vi "Save-images.vi"(8 "error in":errorcluster, 10 "Storage element in":T1 {"Temperature characteristics"."Stand. dev. temperature" format="%#.1f"; "Temperature characteristics"."Min. temperature" format="%#.0f"; "Temperature characteristics"."Max. temperature" format="%#.0f"; "Temperature characteristics"."Average temperature" format="%#.0f"}, 11 "Storage params. ref.":refnum<data-value>) -> (0 "error IO":errorcluster, 2 "Storage element":T1 {"Temperature characteristics"."Stand. dev. temperature" format="%#.1f"; "Temperature characteristics"."Min. temperature" format="%#.0f"; "Temperature characteristics"."Max. temperature" format="%#.0f"; "Temperature characteristics"."Average temperature" format="%#.0f"}, 3 "Storage params. ref.":refnum<data-value>)   [LabVIEW 2013, in "CameraVision.lvlib" / "CV-Main.lvclass"]
uses:
  CV-Main.lvclass
  Storage/CV-Storage.lvclass
  Buffers/Storage-buffer.ctl
  <vilib>/vision/Image Controls.llb/IMAQ Image.ctl
  Temperature/Temperature-characteristics.ctl
  Analysis/Characteristics-cluster.ctl
  Storage/CV-Storage.lvclass/CV-Storage.ctl
  Storage/Read Storage directory.vi
  Storage/Read Save what.vi
  Storage/Read Storage labels.vi
  Storage/Read Storage prefix.vi
  Storage/Read Image file type.vi
  Storage/Read Camera suffix.vi
  Storage/Save-image-with-right-filetype.vi
  Temperature/CV-Temperature.lvclass
  Analysis/CV-Analysis.lvclass
  Buffers/CV-Buffers.lvclass
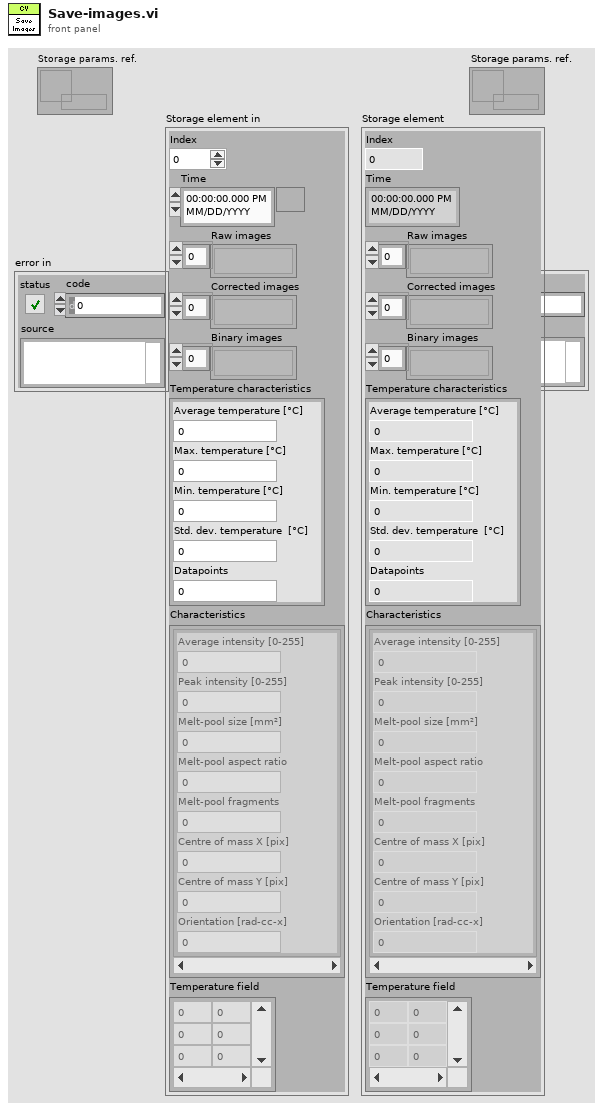
[diagram p1: front panel]
types:
  T1 = typedef "CameraVision.lvlib/CV-Buffers.lvclass/Storage-buffer.ctl" = cluster{"Index":i32, "Time":timestamp, "Raw images":T2[], "Corrected images":T2[], "Binary images":T2[], "Temperature characteristics":T3, "Characteristics":T4[], "Temperature field":dbl[][]}
  T2 = typedef "IMAQ Image.ctl" = refnum<image>
  T3 = typedef "CameraVision.lvlib/CV-Temperature.lvclass/Temperature-characteristics.ctl" = cluster{"Average temperature ":dbl, "Max. temperature":dbl, "Min. temperature":dbl, "Stand. dev. temperature":dbl, "Datapoints":dbl}
  T4 = typedef "CameraVision.lvlib/CV-Analysis.lvclass/Characteristics-cluster.ctl" = cluster{"Average intensity":dbl, "Peak intensity":dbl, "Melt-pool size":dbl, "Melt-pool aspect ratio":dbl, "Melt-pool fragments":dbl, "Centre of mass X":dbl, "Centre of mass Y":dbl, "Orientation":dbl}
  T5 = cluster{"Original":bool, "Corrected":bool, "Binary":bool, "Temperature":bool, "Characteristics":bool, "Mapping":bool, "TemperatureValues":bool}
  T6 = typedef "CameraVision.lvlib/Storage.lvclass/Storage-types-labels.ctl" = cluster{"Original":string, "Corrected":string, "Binary":string, "Temperature":string, "Characteristics":string, "Mapping":string, "TemperatureValues":string}
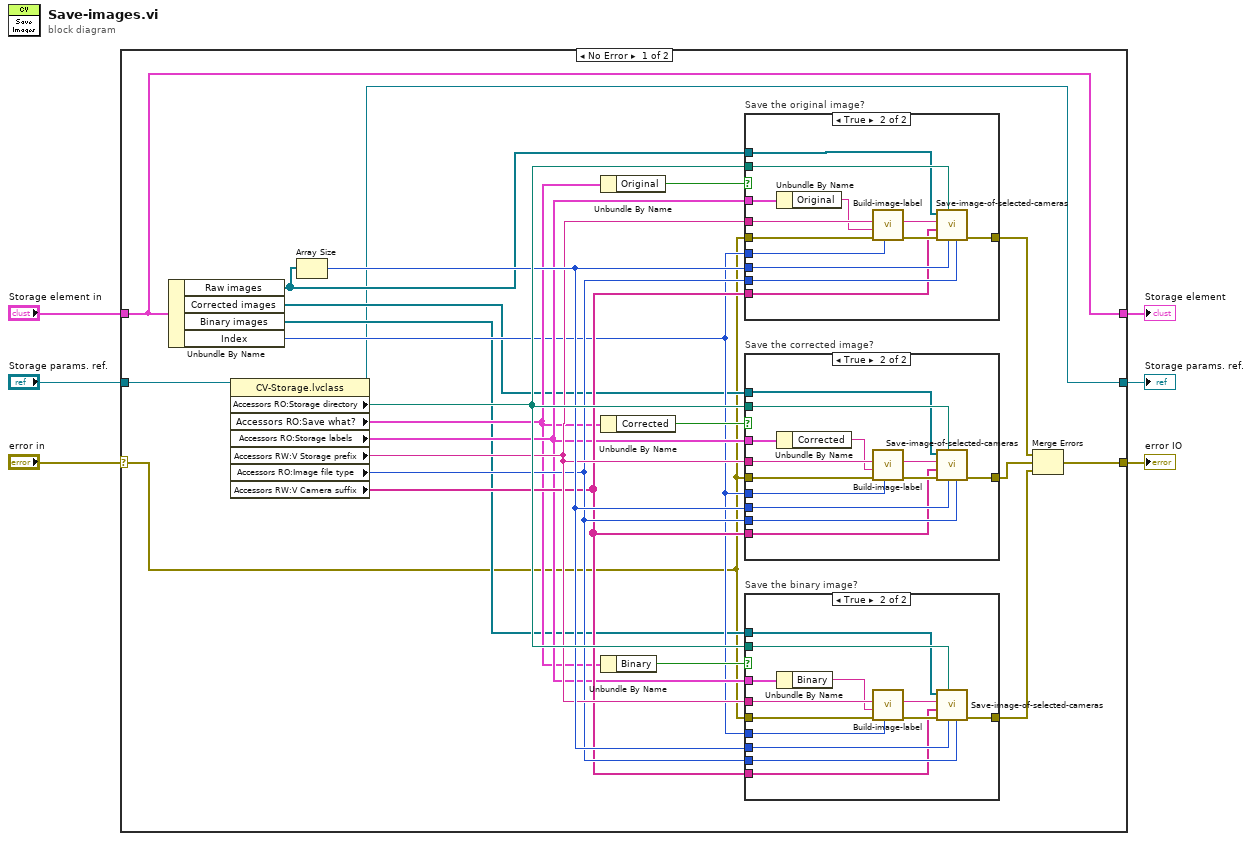
[diagram p0: block diagram]
diagram:
  n1 = case shown="No Error" "error in" {
    selector: "error in" -> [w11 w73]
    tunnel: [w7 w73] -> w6
    tunnel: "Storage params. ref." -> [w25 w72]
    tunnel: "Storage element in" -> [w9 w71]
    tunnel: [w9 w71] -> w2
    tunnel: [w8 w72] -> w1
    frame No Error {
      n2 = Unbundle By Name(w9) -> ("Raw images"=w10:T2[], "Corrected images"=w12:T2[], "Binary images"=w13:T2[], "Index"=w14:i32)
      n3 = property class="CV-Storage.lvclass"(reference=w25) -> (reference out=w8:refnum<data-value>, "Accessors RO:Storage directory"=w28:path, "Accessors RO:Save what?"=w21:T5, "Accessors RO:Storage labels"=w22:T6, "Accessors RW:V Storage prefix"=w26:string, "Accessors RO:Image file type"=w24:enum16{"JPG", "BMP", "PNG"}, "Accessors RW:V Camera suffix"=w23:string[])  [unwired: 1 in, 1 out]
      n4 = Array Size(array=w10) -> (size(s)=w27:i32)
      n5 = Unbundle By Name(w21) -> ("Original"=w20:bool)
      n6 = Unbundle By Name(w21) -> ("Corrected"=w19:bool)
      n7 = Unbundle By Name(w21) -> ("Binary"=w18:bool)
      n8 = case "Save the original image?" shown="True" w20 {
        tunnel: w14 -> [_ w62]
        tunnel: w11 -> [w57 w64]
        tunnel: w10 -> [_ w58]
        tunnel: w28 -> [_ w68]
        tunnel: w27 -> [_ w63]
        tunnel: w26 -> [_ w67]
        tunnel: w22 -> [_ w66]
        tunnel: w24 -> [_ w61]
        tunnel: w23 -> [_ w60]
        tunnel: [w57 w59] -> w17
        frame False {
        }
        frame True {
          n9 = Unbundle By Name(w66) -> ("Original"=w65:string)
          n10 = call "Build-image-label.vi"("Image #"=w62, "error in"=w64, "Image label"=w65, "Base file name"=w67) -> ("error IO"=w69:errorcluster, "Filename"=w70:string)  [unwired: 6 in]
          n11 = call "Save-image-of-selected-cameras.vi"("Image file type"=w61, "Cameras"=w63, "Storage directory"=w68, "error in"=w69, "Camera suffix"=w60, "Filename"=w70, "Image references"=w58) -> ("error IO"=w59:errorcluster)  [unwired: 4 in]
        }
      }
      n12 = case "Save the corrected image?" shown="True" w19 {
        tunnel: w14 -> [_ w48]
        tunnel: w11 -> [w43 w50]
        tunnel: w12 -> [_ w44]
        tunnel: w28 -> [_ w54]
        tunnel: w27 -> [_ w49]
        tunnel: w26 -> [_ w53]
        tunnel: w22 -> [_ w52]
        tunnel: w24 -> [_ w47]
        tunnel: w23 -> [_ w46]
        tunnel: [w43 w45] -> w16
        frame False {
        }
        frame True {
          n13 = Unbundle By Name(w52) -> ("Corrected"=w51:string)
          n14 = call "Build-image-label.vi"("Image #"=w48, "error in"=w50, "Image label"=w51, "Base file name"=w53) -> ("error IO"=w55:errorcluster, "Filename"=w56:string)  [unwired: 6 in]
          n15 = call "Save-image-of-selected-cameras.vi"("Image file type"=w47, "Cameras"=w49, "Storage directory"=w54, "error in"=w55, "Camera suffix"=w46, "Filename"=w56, "Image references"=w44) -> ("error IO"=w45:errorcluster)  [unwired: 4 in]
        }
      }
      n16 = case "Save the binary image?" shown="True" w18 {
        tunnel: w14 -> [_ w34]
        tunnel: w11 -> [w29 w36]
        tunnel: w13 -> [_ w30]
        tunnel: w28 -> [_ w40]
        tunnel: w27 -> [_ w35]
        tunnel: w26 -> [_ w39]
        tunnel: w22 -> [_ w38]
        tunnel: w24 -> [_ w33]
        tunnel: w23 -> [_ w32]
        tunnel: [w29 w31] -> w15
        frame False {
        }
        frame True {
          n17 = Unbundle By Name(w38) -> ("Binary"=w37:string)
          n18 = call "Build-image-label.vi"("Image #"=w34, "error in"=w36, "Image label"=w37, "Base file name"=w39) -> ("error IO"=w41:errorcluster, "Filename"=w42:string)  [unwired: 6 in]
          n19 = call "Save-image-of-selected-cameras.vi"("Image file type"=w33, "Cameras"=w35, "Storage directory"=w40, "error in"=w41, "Camera suffix"=w32, "Filename"=w42, "Image references"=w30) -> ("error IO"=w31:errorcluster)  [unwired: 4 in]
        }
      }
      n20 = Merge Errors(w17, w16, w15) -> (w7:errorcluster)
    }
    frame Error {
    }
  }
  "error IO" <- w6
  "Storage element" <- w2
  "Storage params. ref." <- w1
